vi "lp-server-events.vi"() -> ()   [LabVIEW 2019]
uses:
  vi.lib/addons/zeromq/socket_type.ctl
  vi.lib/addons/zeromq/zmq_context.lvclass
  vi.lib/addons/zeromq/zeromq.lvlib
  vi.lib/addons/zeromq/zmq_socket.lvclass
panel:
  out "element":string
  out "time (ms)":u32
  in  "stop?":bool
  in  "endpoint":string="tcp://127.0.0.1:5555"
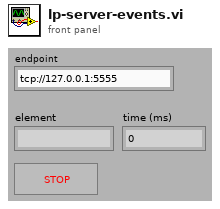
[diagram p1: front panel]
types:
  T1 = typedef "zeromq.lvlib/socket_type.ctl" = enum8{"ZMQ_PAIR", "ZMQ_PUB", "ZMQ_SUB", "ZMQ_REQ", "ZMQ_REP", "ZMQ_DEALER", "ZMQ_ROUTER", "ZMQ_PULL", "ZMQ_PUSH", "ZMQ_XPUB", "ZMQ_XSUB"}
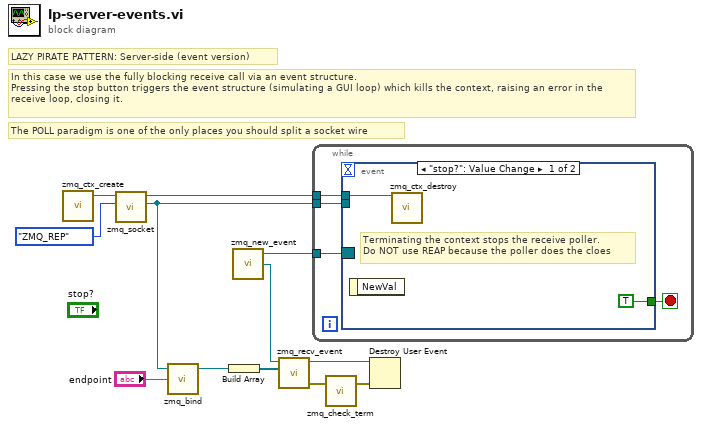
[diagram p0: block diagram]
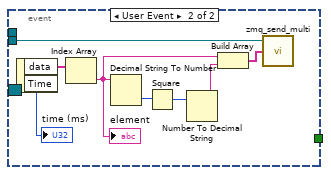
[diagram p2: hidden frame]
diagram:
  # "The POLL paradigm is one of the only places you should split a socket wire"
  # "In this case we use the fully blocking receive call via an event structure.\nPressing the stop button triggers the event structure (simulating a GUI loop) which kills the context, raising an error in the receive loop, closing it."
  # "LAZY PIRATE PATTERN: Server-side (event version)"
  n1 = call "zmq_ctx_create.vi"() -> ("context out"=w10:refnum<class "zmq_context.lvclass">)  [unwired: 4 in, 1 out]
  n2 = call "zmq_socket.vi"("socket type"=socket_type."ZMQ_REP", "context in"=w10) -> ("socket out"=w5:refnum<class "zmq_socket.lvclass">, "context out"=w9:refnum<class "zmq_context.lvclass">)  [unwired: 3 in, 1 out]
  n3 = call "zmq_bind.vi"("endpoint"="endpoint", "socket in"=w5) -> ("socket out"=w4:refnum<class "zmq_socket.lvclass">)  [unwired: 2 in, 1 out]
  n4 = Build Array(w4) -> (w8:refnum<class "zmq_socket.lvclass">[])
  n5 = call "zmq_new_event.vi"() -> ("user event"=w6:refnum<user-event>, "event ref out"=w7:refnum<event-registration>)  [unwired: 3 in, 1 out]
  n6 = call "zmq_recv_event.vi"("sockets"=w8, "poll event"=w6) -> ("error out"=w3:errorcluster, "poll event out"=w2:refnum<user-event>)  [unwired: 4 in]
  n7 = while {
    tunnel: w9 -> [w16]
    tunnel: w7 -> [w15]
    tunnel: w5 -> [w13]
    stop <- w14 stop-if-true
    n8 = event shown="[0] \"stop?\": Value Change" {
      selector: w15 -> [_ _]
      dyn-events: _ -> [_ _]
      timeout: _ -> [_ _]
      tunnel: w16 -> [w18 _]
      tunnel: w13 -> [_ w20]
      tunnel: [TRUE ("NewVal") _] -> w14
      event "stop?": Value Change {
        # "Terminating the context stops the receive poller.\nDo NOT use REAP because the poller does the cloes"
        n9 = event-data() -> ()  [unwired: 1 in, 1 out]
        n10 = call "zmq_ctx_destroy.vi"("context in"=w18) -> ()  [unwired: 4 in, 1 out]
      }
      event User Event {
        n11 = event-data() -> ("data"=w22:string[], "Time"=→"time (ms)":u32)  [unwired: 1 in]
        n12 = Index Array(array=w22) -> (element=w21:string)  [unwired: 1 in]
        "element" <- w21
        n13 = Decimal String To Number(string=w21) -> (number=w23:i32)  [unwired: 2 in, 1 out]
        n14 = Square(x=w23) -> (x^2=w24:i32)
        n15 = Number To Decimal String(number=w24) -> (decimal integer string=w25:string)  [unwired: 1 in]
        n16 = Build Array(w21, w25) -> (w26:string[])
        n17 = call "zmq_send_multi.vi"("parts"=w26, "socket in"=w20) -> ()  [unwired: 2 in, 2 out]
      }
    }
  }
  n18 = call "zmq_check_term.vi"("error in"=w3) -> ("error out"=w1:errorcluster)  [unwired: 1 in, 1 out]
  n19 = Destroy User Event(user event=w2, error in=w1) -> ()  [unwired: 1 out]
